vi "Map.vi"() -> ()   [LabVIEW 2010]
uses:
  Utilities/Waypoint.ctl
  Utilities/ModemTelemetryPacket.ctl
  <vilib>/Utility/sysdir.llb/System Directory Type.ctl
  <vilib>/Utility/config.llb/Write Key (String).vi
  <vilib>/Utility/config.llb/Read Key (String).vi
  <vilib>/Utility/config.llb/NI_LVConfig.lvlib
panel:
  in  "Map":refnum<k7>(container)
  out "HDOP":u16
  out "Sat Count":u16
  in  "Update Rate":dbl=5.0
  out "RSSI":u8(slide) scale=0.0..100.0
  out "Heading":u32(colorbox)=16448250
  out "Course":u32(colorbox)
  out "Capacity":u16
  out "Heading":i16
  out "Course":i16
  out "Speed":u8
  out "Altitude":dbl format="%#.1f"
  out "Longitude":dbl
  out "Latitude":dbl
  out "Battery":dbl(slide) scale=9.0..12.0 scale format="%.1f"
  out "Current":u8
  out "Voltage":dbl
  out "Compass":cluster{dbl, dbl}(knob)={0.0, 51.49737856172287} scale=0.0..360.0
  in  "Slider":bool
  out "VehiclePositionState":bool
  in  "VehicleUpdate":bool
  in  "Center":bool
  in  "Recall":bool
  in  "Load":bool
  in  "Save":bool
  in  "NoFly":bool
  in  "Home":bool
  in  "Waypoint List":T1[](array[typedef]) {"EW" items=["E", "W"]; "LonS" format="%#.1f"; "NS" items=["N", "S"]; "LatS" format="%#.1f"}
  in  "ManualAdd":bool
  in  "Up":bool
  in  "Down":bool
  in  "Delete":bool
  in  "Clear":bool
  in  "Upload":bool
  # "Lattitude"
  # "Longitude"
  # "Altitude"
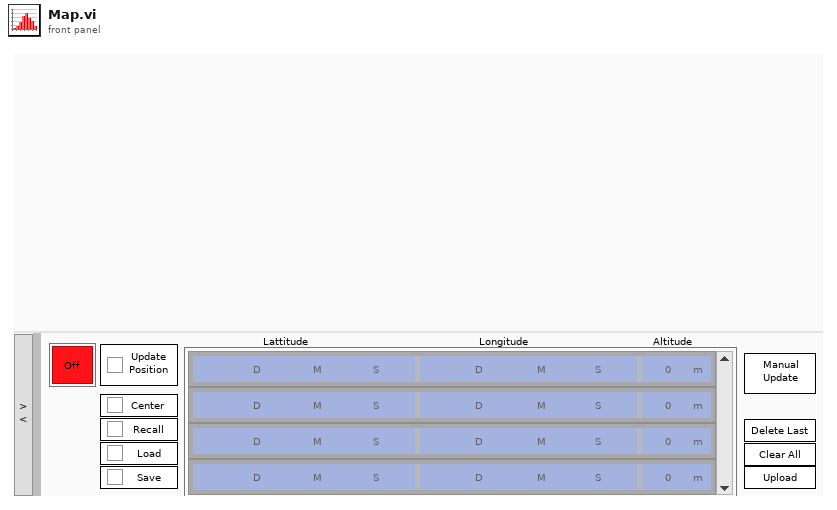
[diagram p1: front panel]
types:
  T1 = typedef "Waypoint.ctl" = cluster{"LatD":dbl, "LatM":dbl, "LatS":dbl, "LonD":dbl, "LonM":dbl, "LonS":dbl, "Alt":dbl, "NS":u16, "EW":u16}
  T2 = cluster{"Error":errorcluster, "GUIQueue":refnum<queue>, "IniData":string[][], "Map":refnum<k7>, "CookiePath":path, "Waypoints":T1[], "LastAlt":dbl, "LastType":u16, "Data":i32[][], "TlmType":string, "Compare":i32[], "Null":T1[], "MaxWaypoints":i32, "InvalidAngle":i32, "InvalidAltitude":i32, "Previous":string, "Retry":i32, "ModemQueue":refnum<queue>, "Internet":bool}
  T3 = typedef "LVRectTypeDef.ctl" = cluster{"left":i16, "top":i16, "right":i16, "bottom":i16}
  T4 = enum32{"invalid app kind", "Development System", "Run Time System", "Student Edition", "Embedded LabVIEW", "Evaluation", "Custom"}
  T5 = typedef "System Directory Type.ctl" = i32
  T6 = typedef "NI_LVConfig.lvlib/Config Data RefNum.ctl" = refnum<k1>
  T7 = enum8{"Enabled", "Disabled", "Disabled and Grayed Out"}
  T8 = typedef "ModemTelemetryPacket.ctl" = cluster{"id":u16, "latitude":i32, "longitude":i32, "altitude":i16, "course":i16, "heading":i16, "speed":u8, "voltage":u8, "current":u8, "capacity":u16, "reserved":u16, "ecc":u8[], "RSSI":u8}
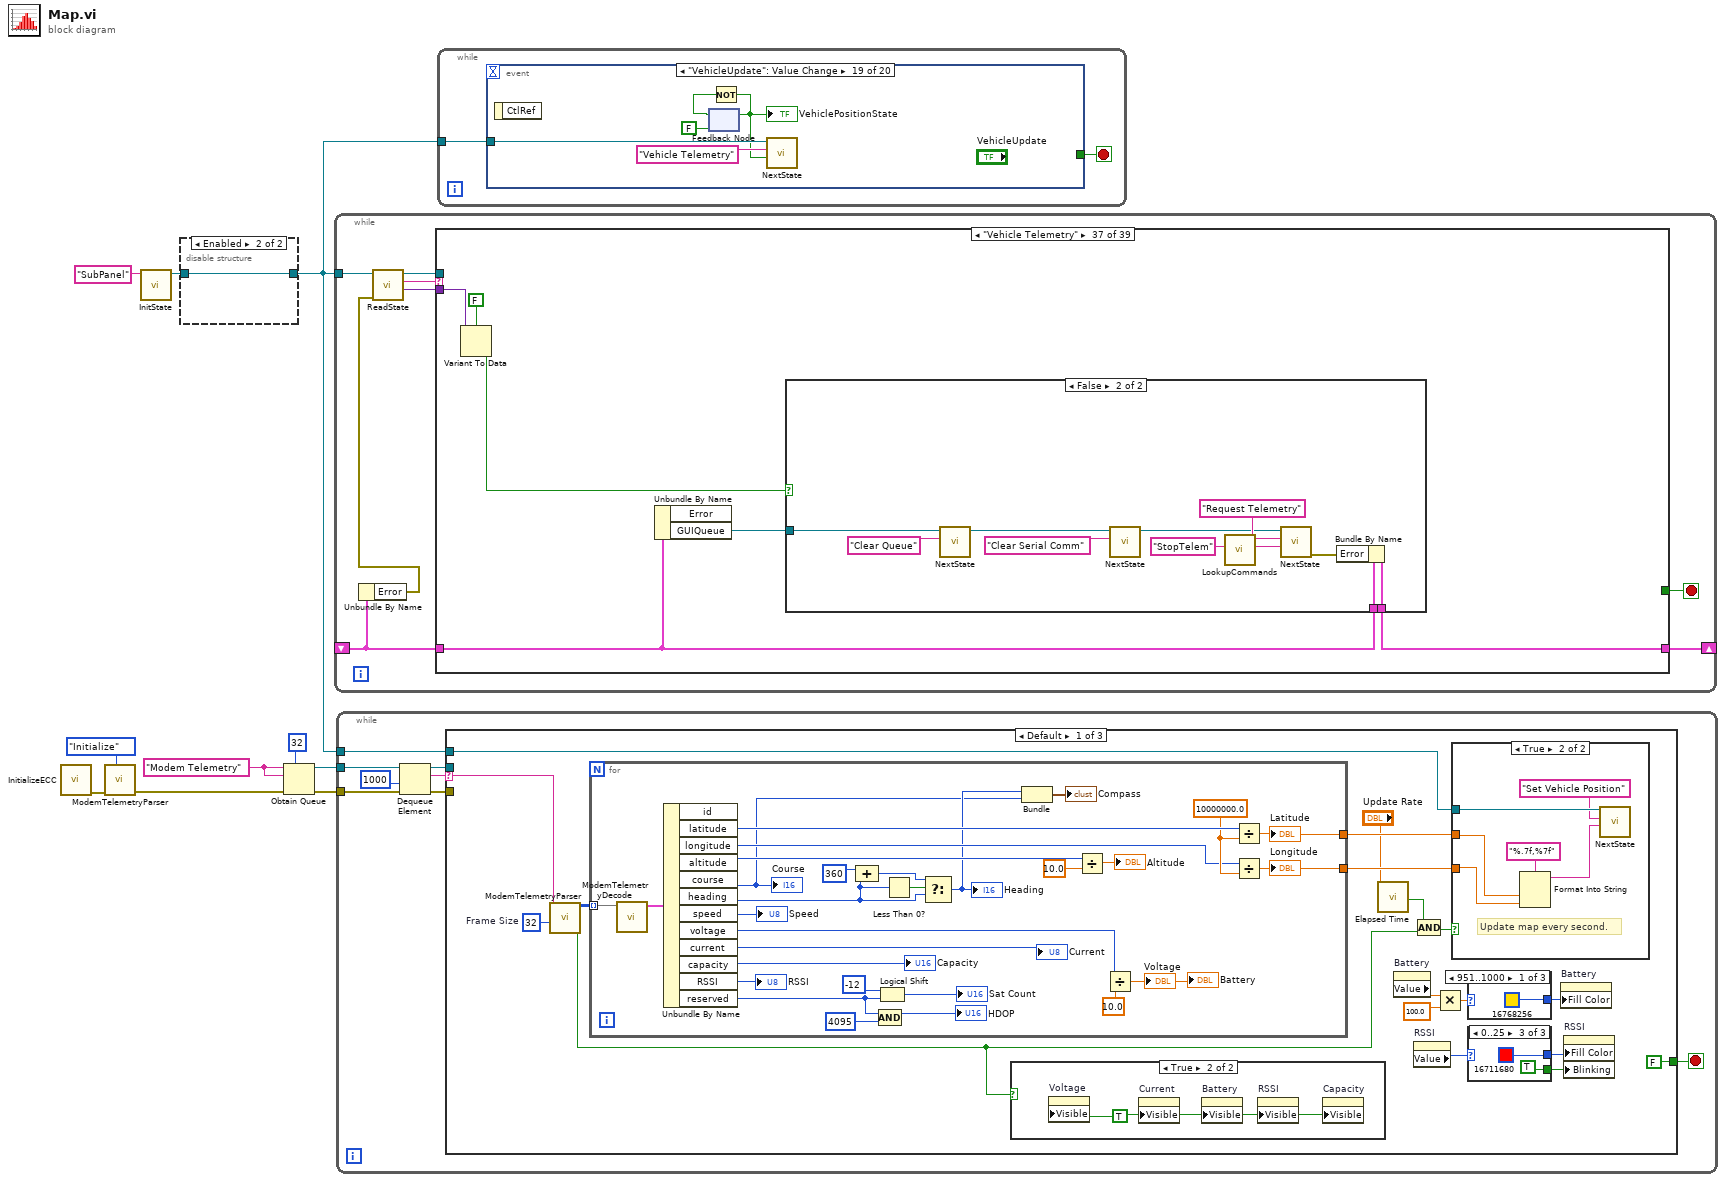
[diagram p0: block diagram]
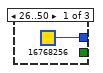
[diagram p3: hidden frame]
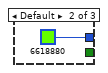
[diagram p4: hidden frame]
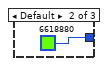
[diagram p5: hidden frame]
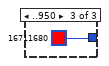
[diagram p6: hidden frame]
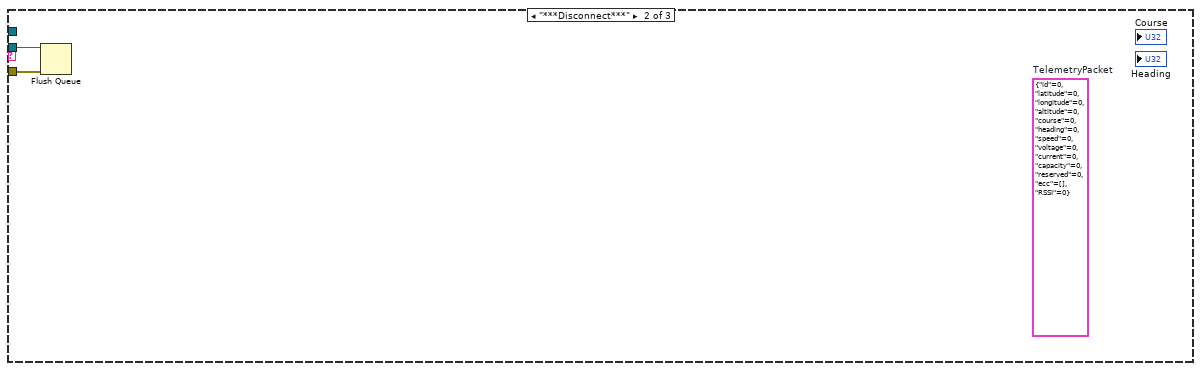
[diagram p8: hidden frame]
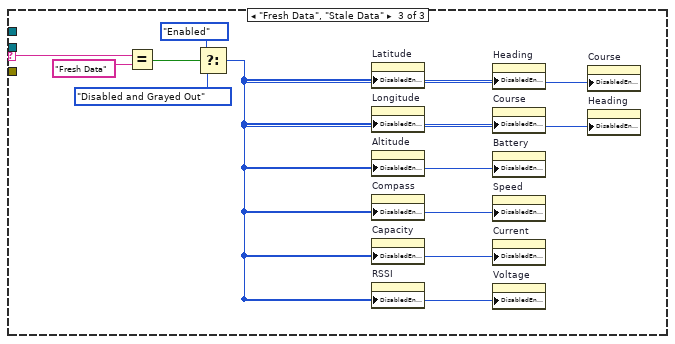
[diagram p9: hidden frame]
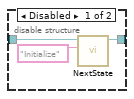
[diagram p10: hidden frame]
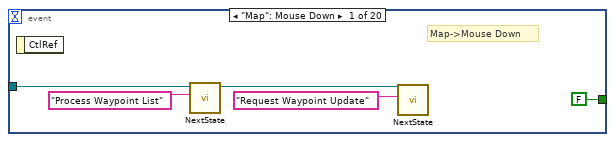
[diagram p11: hidden frame]
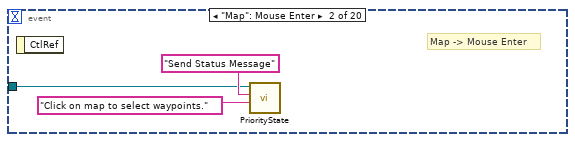
[diagram p12: hidden frame]
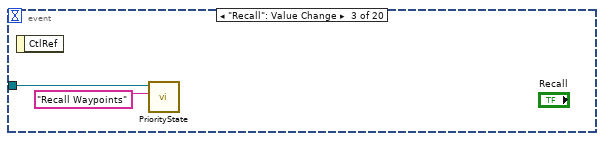
[diagram p13: hidden frame]
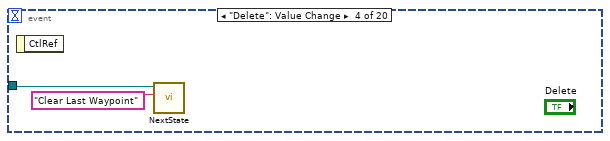
[diagram p14: hidden frame]
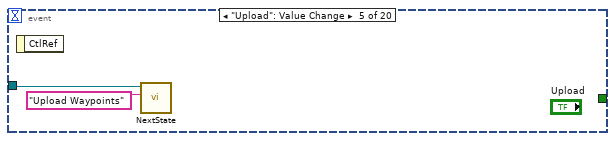
[diagram p15: hidden frame]
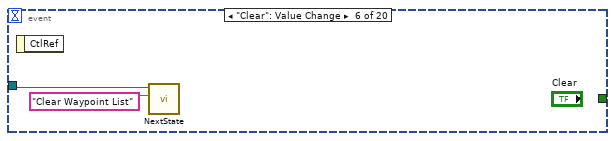
[diagram p16: hidden frame]
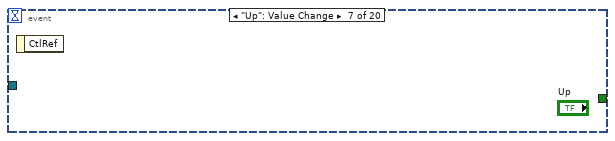
[diagram p17: hidden frame]
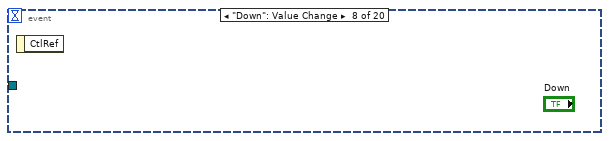
[diagram p18: hidden frame]
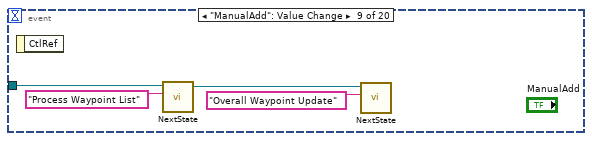
[diagram p19: hidden frame]
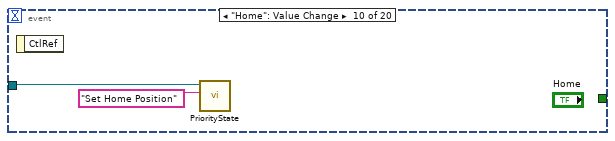
[diagram p20: hidden frame]
diagram:
  w6 = "Modem Telemetry" ("name (unnamed)")
  n1 = call "InitializeECC.vi"() -> ("Error Out"=w5:errorcluster)  [unwired: 11 in]
  n2 = call "ModemTelemetryParser.vi"("Operation"=enum16{"Parse", "Initialize"}."Initialize", "Error In"=w5) -> ("Error Out"=w4:errorcluster)  [unwired: 7 in, 2 out]
  n3 = call "InitState.vi"("Name"="SubPanel" ("name (unnamed)")) -> ("Queue Out"=w9:refnum<queue>)  [unwired: 8 in, 1 out]
  n4 = disable-structure shown="Enabled" {
    disable-tunnel: w9 -> [w13 w14]
    disable-tunnel: [w12 w14] -> w8
    frame Disabled {
      n5 = call "NextState.vi"("State"="Initialize", "Queue In"=w13) -> ("Queue Out"=w12:refnum<queue>)  [unwired: 8 in, 1 out]
    }
    frame Enabled {
    }
  }
  n6 = Obtain Queue(max queue size (-1, unlimited)=32, name (unnamed)=w6, element data type=w6, error in (no error)=w4) -> (queue out=w2:refnum<queue>, error out=w1:errorcluster)  [unwired: 1 in, 1 out]
  n7 = while {
    tunnel: w8 -> [w18]
    shift-right: [w22] -> _
    shift-left: _ -> [w21]
    stop <- w20 stop-if-true
    n8 = Unbundle By Name(w21) -> ("Error"=w19:errorcluster)
    n9 = call "ReadState.vi"("Error In"=w19, "Queue In"=w18) -> ("Data"=w15:variant, "State"=w17:string, "Queue Out"=w16:refnum<queue>)  [unwired: 6 in, 1 out]
    n10 = case shown="\"Vehicle Telemetry\"" w17 {
      tunnel: [w23 w25 w47 w55 w61 w69 w74 w98 w115 w118 w127 w128 w132 w148 w185 w200 w206 w211 w217 w227 w245 w289 w319 w334 w385 w391 w409 w421 w489 w505 w562 w572 w585 w587 w639 w721 w726 w756 w790] -> w22
      tunnel: w21 -> [w23 w25 _ w55 w62 w69 w74 w98 w115 w118 w127 w128 w132 w149 w173 w200 w206 w212 w217 w225 w245 w288 w319 w335 w385 w392 w410 w422 w489 w506 w563 w572 w585 w588 w638 w721 w727 w756 w790]
      tunnel: [_ TRUE _ _ _ _ _ _ _ _ TRUE _ _ _ _ _ _ _ _ _ _ _ _ _ _ _ _ _ _ _ _ _ _ _ _ _ _ _ _] -> w20
      tunnel: w16 -> [_ _ w42 _ _ _ _ _ _ _ _ _ w133 w156 w177 w201 _ w210 _ w223 w246 _ w321 _ w386 w394 _ w420 _ w509 _ _ _ _ w636 _ _ w753 _]
      tunnel: w15 -> [_ _ w44 w58 _ w68 _ _ _ _ _ _ _ _ _ _ _ w215 _ _ _ _ _ _ _ _ _ _ _ _ _ _ _ _ _ _ w724 _ w785]
      selector: w17 -> [_ w26 _ w57 _ _ _ _ _ _ _ _ _ _ _ _ _ _ _ _ _ _ _ _ _ _ w407 _ _ _ _ _ _ _ _ _ _ _ w786]
      frame "--- System ---" {
      }
      frame Default {
        n11 = Format Into String(format string="Invalid state:\n%s", w26) -> (resulting string=w27:string)  [unwired: 2 in, 1 out]
        n12 = One Button Dialog(message=w27) -> ()  [unwired: 1 in, 1 out]
      }
      frame "Initialize" {
        w40 = T1[] []  # Waypoints
        w37 = T2 {"Error"={"status"=FALSE, "code"=0, "source"=""}, "GUIQueue"=refnum, "IniData"=[], "Map"=refnum, "CookiePath"=path "", "Waypoints"=[], "LastAlt"=5.0, "LastType"=0, "Data"=[], "TlmType"="", "Compare"=[], "Null"=[], "MaxWaypoints"=16, "InvalidAngle"=2147483647, "InvalidAltitude"=999999999, "Previous"="", "Retry"=3, "ModemQueue"=refnum, "Internet"=FALSE}
        n13 = Variant To Data(Variant=w44, type=string[][] [] ("subarray")) -> (data=w29:string[][])  [unwired: 1 in, 1 out]
        n14 = Build Array(0) -> (w39:i32[])
        n15 = property on="Waypoint List" class="Arr (strict)"("Index Values"=w39) -> ()  [unwired: 2 in, 2 out]
        n16 = Unbundle By Name(w37) -> ("InvalidAngle"=w33:i32, "InvalidAltitude"=w32:i32, "MaxWaypoints"=w36:i32)
        n17 = call "NextStates.vi"("States"=string[] ["Read Initialization"], "Queue In"=w42) -> ()  [unwired: 8 in, 2 out]
        n18 = Bundle By Name(cluster=T1 {"LatD"=2147483647.0, "LatM"=2147483647.0, "LatS"=2147483647.0, "LonD"=2147483647.0, "LonM"=2147483647.0, "LonS"=2147483647.0, "Alt"=999999999.0, "NS"=0, "EW"=0} ("Waypoint"), "LatD"=w33, "LatM"=w33, "LatS"=w33, "LonD"=w33, "LonM"=w33, "LonS"=w33, "Alt"=w32) -> (w31:T1)
        n19 = Initialize Array(w31, w36) -> (w35:T1[])
        n20 = property class="App"() -> ("OS.Version"=w43:string)  [unwired: 2 in, 2 out]
        n21 = case shown="\"5.1\"" w43 {
          tunnel: [_ w49 w52] -> w30
          frame Default {
          }
          frame "5.1" {
            n22 = Temporary Directory() -> (w51:path)
            n23 = Build Path(base path=w51, name or relative path="..\\..\\..\\Cookies") -> (appended path=w49:path)
          }
          frame "6.1" {
            n24 = Temporary Directory() -> (w53:path)
            n25 = Build Path(base path=w53, name or relative path="..\\..\\Roaming\\Microsoft\\Windows\\Cookies") -> (appended path=w52:path)
          }
        }
        n26 = call "InitState.vi"("Name"="GUI") -> ("Queue Out"=w45:refnum<queue>)  [unwired: 8 in, 1 out]
        n27 = Bundle By Name(cluster=w37, "CookiePath"=w30, "GUIQueue"=w45, "IniData"=w29, "Null"=w35) -> (w47:T2)
        n28 = local write "Waypoint List"(w40) -> ()
      }
      frame "Send Status Message" {
        n29 = Unbundle By Name(w55) -> ("GUIQueue"=w59:refnum<queue>)
        n30 = Variant To Data(Variant=w58, type=w57) -> (data=w56:string)  [unwired: 1 in, 1 out]
        n31 = call "NextState.vi"("Data"=w56, "State"="Status", "Queue In"=w59) -> ()  [unwired: 7 in, 2 out]
      }
      frame "Error" {
        n32 = Unbundle By Name(w62) -> ("Error"=w65:errorcluster)
        n33 = call "ErrorDialog.vi"("error in"=w65) -> ("error out"=w64:errorcluster)  [unwired: 10 in]
        n34 = call <vilib>:"Clear Errors.vi"("error in (no error)"=w64) -> ("error out"=w63:errorcluster)  [unwired: 6 in]
        n35 = Bundle By Name(cluster=w62, "Error"=w63) -> (w61:T2)
      }
      frame "Delay" {
        n36 = Variant To Data(Variant=w68, type=0) -> (data=w66:i32)  [unwired: 1 in, 1 out]
        n37 = Wait (ms)(milliseconds to wait=w66) -> ()  [unwired: 1 out]
      }
      frame "Center Map" {
        n38 = Unbundle By Name(w74) -> ("Map"=w75:refnum<k7>, "Waypoints"=w72:T1[])
        n39 = Index Array(array=w72) -> (element=w73:T1)  [unwired: 1 in]
        n40 = Array Size(array=w72) -> (size(s)=w71:i32)
        n41 = Equal To 0?(x=w71) -> (x = 0?=w70:bool)
        n42 = case shown="False" w70 {
          tunnel: w75 -> [w96 _]
          tunnel: w73 -> [w79 _]
          frame False {
            n43 = Unbundle By Name(w79) -> ("NS"=w93:u16, "LatD"=w91:dbl, "LatM"=w88:dbl, "LatS"=w87:dbl, "EW"=w84:u16, "LonD"=w82:dbl, "LonM"=w81:dbl, "LonS"=w80:dbl)
            n44 = Greater Than 0?(x=w84) -> (x > 0?=w86:bool)
            n45 = Greater Than 0?(x=w93) -> (x > 0?=w92:bool)
            n46 = Negate(x=w91) -> (-x=w90:dbl)
            n47 = Negate(x=w82) -> (-x=w83:dbl)
            n48 = Select(t=w90, s=w92, f=w91) -> (s? t:f=w89:dbl)
            n49 = Select(t=w83, s=w86, f=w82) -> (s? t:f=w85:dbl)
            n50 = call "ConvertDMS2DD.vi"("Seconds"=w87, "Minutes"=w88, "Degrees"=w89) -> ("Degree Decimal"=w78:dbl)  [unwired: 7 in, 1 out]
            n51 = call "ConvertDMS2DD.vi"("Seconds"=w80, "Minutes"=w81, "Degrees"=w85) -> ("Degree Decimal"=w77:dbl)  [unwired: 7 in, 1 out]
            n52 = Format Into String(format string="javascript:centerMap(%f,%f,%d);" ("URL"), w78, w77, 17) -> (resulting string=w94:string)  [unwired: 2 in, 1 out]
            n53 = call "WaitForBrowser.vi"("BrowserCommand"=w94, "BrowserRef"=w96) -> ()  [unwired: 8 in, 2 out]
          }
          frame True {
            n54 = One Button Dialog(message="No waypoints found!  Please try loading waypoints to the AeroQuad first.") -> ()  [unwired: 1 in, 1 out]
          }
        }
      }
      frame "Move Slider" {
        n55 = property class="VI"() -> ("Front Panel.PanelBounds"=w113:T3)  [unwired: 2 in, 2 out]
        n56 = Unbundle By Name(w113) -> ("right"=w111:i16, "left"=w112:i16)
        n57 = Subtract(x=w111, y=w112) -> (x-y=w108:i16)
        n58 = property on="Splitter 5" class="Splitter"() -> ("Width"=w105:u32)  [unwired: 2 in, 2 out]
        n59 = property on="Splitter 5" class="Splitter"() -> ("Position"=w109:i32)  [unwired: 2 in, 2 out]
        n60 = property on="Slider" class="Bool"() -> ("Width"=w101:u32)  [unwired: 2 in, 2 out]
        n61 = To Unsigned Long Integer(number=w108) -> (unsigned 32bit integer=w104:u32)
        n62 = Increment(x=w105) -> (x+1=w103:u32)
        n63 = Divide(x=w108, y=2.0) -> (x/y=w106:dbl)
        n64 = Increment(x=w101) -> (x+1=w100:u32)
        n65 = Greater Or Equal?(x=w109, y=w106) -> (x >= y?=w107:bool)
        n66 = Subtract(x=w104, y=w103) -> (x-y=w102:u32)
        n67 = Select(t=w100, s=w107, f=w102) -> (s? t:f=w99:u32)
        n68 = property on="Splitter 5" class="Splitter"("Position"=w99) -> ()  [unwired: 2 in, 2 out]
      }
      frame "Move Slider Waypoint" {
        n69 = property on="Slider" class="Bool"() -> ("Width"=w116:u32)  [unwired: 2 in, 2 out]
        n70 = Increment(x=w116) -> (x+1=w114:u32)
        n71 = property on="Splitter 5" class="Splitter"("Position"=w114) -> ()  [unwired: 2 in, 2 out]
      }
      frame "Move Slider Modem" {
        n72 = property class="VI"() -> ("Front Panel.PanelBounds"=w125:T3)  [unwired: 2 in, 2 out]
        n73 = Unbundle By Name(w125) -> ("right"=w123:i16, "left"=w124:i16)
        n74 = Subtract(x=w123, y=w124) -> (x-y=w122:i16)
        n75 = property on="Splitter 5" class="Splitter"() -> ("Width"=w121:u32)  [unwired: 2 in, 2 out]
        n76 = To Unsigned Long Integer(number=w122) -> (unsigned 32bit integer=w120:u32)
        n77 = Increment(x=w121) -> (x+1=w119:u32)
        n78 = Subtract(x=w120, y=w119) -> (x-y=w117:u32)
        n79 = property on="Splitter 5" class="Splitter"("Position"=w117) -> ()  [unwired: 2 in, 2 out]
      }
      frame "Shutdown" {
      }
      frame "--- Setup ---" {
      }
      frame "Read Initialization" {
        w131 = string[] ["WaypointList", "WaypointVerify", "WriteEEPROM", "Telemetry", "StopTelem"]
        n80 = Unbundle By Name(w132) -> ("IniData"=w138:string[][], "GUIQueue"=w137:refnum<queue>)
        n81 = call "NextState.vi"("State"="Check Internet", "Queue In"=w133) -> ()  [unwired: 8 in, 2 out]
        n82 = call "NextState.vi"("Data"="Click on map to select waypoints." ("State"), "State"="Status", "Queue In"=w137) -> ()  [unwired: 7 in, 2 out]
        n83 = Index Array(array=w138, index (col)=0 ("index (row)")) -> (element=w140:string[])  [unwired: 1 in]
        n84 = for {
          tunnel: w140 -> [w146]
          tunnel: w131 -> [w142] mode=indexing
          tunnel: w138 -> [w145]
          tunnel: [w141] -> w130 mode=indexing
          n85 = Search 1D Array(1D array=w146, element=w142) -> (index of element=w143:i32)  [unwired: 1 in]
          n86 = Index Array(array=w145, index (row)=w143, index (col)=1 ("disabled index (col)")) -> (element=w141:string)
        }
        n87 = call "LookupCommands.vi"("CommandValues"=w130, "CommandNames"=w131, "Mode"=enum16{"Read", "Initialize"}."Initialize") -> ()  [unwired: 8 in, 1 out]
      }
      frame "Check Internet" {
        w155 = "74.125.127.95"  # maps.googleapis.com
        n88 = TCP Open Connection(address=w155, remote port or service name=u16 80, timeout ms (60000)=3000) -> (connection ID=w151:refnum<k5>, error out=w152:errorcluster)  [unwired: 2 in]
        n89 = TCP Close Connection(connection ID=w151, error in (no error)=w152) -> (error out=w150:errorcluster)  [unwired: 1 in, 1 out]
        n90 = case shown="No Error" w150 {
          tunnel: w156 -> [w161 w166]
          tunnel: [TRUE ("T button?") w163] -> w147
          frame No Error {
            n91 = call "NextState.vi"("Data"="Searching for stored waypoints..." ("State"), "State"="Send Status Message", "Queue In"=w161) -> ("Queue Out"=w160:refnum<queue>)  [unwired: 7 in, 1 out]
            n92 = call "NextState.vi"("State"="Load Map", "Queue In"=w160) -> ()  [unwired: 8 in, 2 out]
          }
          frame Error {
            n93 = Two Button Dialog(message="This feature requires a network connection.", 1:"Continue" ("T button name (\"OK\")"), 2:"Retry" ("T button name (\"OK\")")) -> (T button?=w163:bool)
            n94 = case shown="True" w163 {
              tunnel: w166 -> [_ w170]
              tunnel: "Check Internet" -> [_ w169]
              frame False {
              }
              frame True {
                n95 = call "NextState.vi"("State"=w169, "Queue In"=w170) -> ()  [unwired: 8 in, 2 out]
              }
            }
          }
        }
        n96 = Bundle By Name(cluster=w149, "Internet"=w147) -> (w148:T2)
      }
      frame "Load Map" {
        (unwired) "Ask User To Recall Waypoints" ("State")
        n97 = call "NextState.vi"("State"="Recall Waypoints", "Queue In"=w177) -> ()  [unwired: 8 in, 2 out]
        n98 = property class="App"() -> ("App.Kind"=w184:T4)  [unwired: 2 in, 2 out]
        n99 = property class="App"() -> ("OS.Name"=w182:string)  [unwired: 2 in, 2 out]
        n100 = call <userlib>:"Current VIs Parent Directory__ogtk.vi"() -> ("Parent Directory (+ Relative)"=w183:path)  [unwired: 5 in]
        n101 = case shown="\"Run Time System\", Default" w184 {
          tunnel: [w190 w198] -> w180
          tunnel: w183 -> [w193 w198]
          tunnel: w182 -> [w191 _]
          frame "Run Time System", Default {
            n102 = case shown="\"Mac OS\"" w191 {
              tunnel: [w195 w197] -> w194
              tunnel: w193 -> [w195 w196]
              frame Default {
              }
              frame "Mac OS" {
                n103 = Strip Path(path=w196) -> (stripped path=w197:path)  [unwired: 1 out]
              }
            }
            n104 = Build Path(base path=w194, name or relative path=path "Support") -> (appended path=w190:path)
          }
          frame "Development System" {
          }
        }
        n105 = Unbundle By Name(w173) -> ("Internet"=w172:bool)
        n106 = Build Path(base path=w180, name or relative path="AeroQuad.cfg") -> (appended path=w181:path)
        n107 = Path To String(path=w181) -> (string=w179:string)
        n108 = call "WaitForBrowser.vi"("Connection"=w172, "BrowserCommand"=w179, "BrowserRef"="Map") -> ("BrowserRefOut"=w175:refnum<k7>)  [unwired: 7 in, 1 out]
        n109 = disable-structure shown="Disabled" {
          disable-tunnel: w175 -> [w188 w189]
          disable-tunnel: [w187 w189] -> w174
          frame Disabled {
            n110 = call "WaitForBrowser.vi"("BrowserCommand"="javascript:showVehicle(true);", "BrowserRef"=w188) -> ("BrowserRefOut"=w187:refnum<k7>)  [unwired: 8 in, 1 out]
          }
          frame Enabled {
          }
        }
        n111 = Bundle By Name(cluster=w173, "Map"=w174) -> (w185:T2)
      }
      frame "Ask User To Recall Waypoints" {
        n112 = Two Button Dialog(message="Would you like to recall waypoints stored in the AeroQuad?\n\nYou must be connected to the AeroQuad to complete this operation.  Waypoints can be recalled at any time by selecting the \"Recall\" button. ") -> (T button?=w202:bool)  [unwired: 2 in]
        n113 = case shown="True" w202 {
          tunnel: w201 -> [_ w204]
          frame False {
          }
          frame True {
            n114 = call "NextState.vi"("State"="Recall Waypoints", "Queue In"=w204) -> ()  [unwired: 8 in, 2 out]
          }
        }
      }
      frame "Set Home Position" {
        n115 = Unbundle By Name(w206) -> ("Map"=w205:refnum<k7>)
        n116 = flat-sequence {
          tunnel: w205 -> [w207]
          frame #0 {
            n117 = invoke class="IWebBrowser2" method="Navigate"(reference=w207, "URL"="javascript:clearMap();") -> ()  [unwired: 6 in, 8 out]
            n118 = One Button Dialog(message="Click on your desired default start position.") -> ()  [unwired: 1 in, 1 out]
          }
          frame #1 {
            # "Retrieve Waypoint"
          }
          frame #2 {
            # "Store to Disk"
          }
          frame #3 {
            # "Center Map"
          }
        }
      }
      frame "Update" {
        # "When initializing for the type of\ncalibration / telemetry, populate\nTlmType with the state where\nthis data will be processed as\nreceived from main Configurator."
        n119 = Variant To Data(Variant=w215, type=i32[][] []) -> (data=w213:i32[][])  [unwired: 1 in, 1 out]
        n120 = Bundle By Name(cluster=w212, "Data"=w213) -> (w211:T2)
        n121 = Unbundle By Name(w211) -> ("TlmType"=w214:string)
        n122 = call "NextState.vi"("State"=w214, "Queue In"=w210) -> ()  [unwired: 8 in, 2 out]
      }
      frame "--- Configure Waypoints ---" {
      }
      frame "Process Waypoint List" {
        n123 = Unbundle By Name(w225) -> ("MaxWaypoints"=w221:i32)
        n124 = Array Size(array="Waypoint List") -> (size(s)=w224:i32)
        n125 = Greater Or Equal?(x=w224, y=w221) -> (x >= y?=w222:bool)
        n126 = Decrement(x=w224) -> (x-1=w218:i32)
        n127 = Index Array(array="Waypoint List", index=w218) -> (element=w219:T1)
        n128 = Unbundle By Name(w219) -> ("Alt"=w220:dbl)
        n129 = case shown="..-1" w218 {
          tunnel: w220 -> [_ w235]
          tunnel: w225 -> [w230 w234]
          tunnel: "Waypoint List" -> [w228 w233]
          tunnel: [w229 w232] -> w227
          frame ..-1 {
            w231 = u16 0  # Future Use
            n130 = Bundle By Name(cluster=w230, "Waypoints"=w228, "LastType"=w231) -> (w229:T2)
          }
          frame Default {
            w236 = u16 0  # Future Use
            n131 = Bundle By Name(cluster=w234, "Waypoints"=w233, "LastType"=w236, "LastAlt"=w235) -> (w232:T2)
          }
        }
        n132 = case shown="False" w222 {
          tunnel: w223 -> [_ w238]
          tunnel: w221 -> [_ w237]
          frame False {
          }
          frame True {
            n133 = Format Into String(format string="Maximum number of %d waypoints has been reached! ", w237) -> (resulting string=w242:string)  [unwired: 2 in, 1 out]
            n134 = call "NextState.vi"("Data"=w242, "State"="Send Status Message" ("format string"), "Queue In"=w238) -> ("Queue Out"=w243:refnum<queue>)  [unwired: 7 in, 1 out]
            n135 = call "NextState.vi"("State"="Clear Last Waypoint", "Queue In"=w243) -> ()  [unwired: 8 in, 2 out]
          }
        }
      }
      frame "Manual Waypoint Update" {
        n136 = local read "Waypoint List"() -> (w249:T1[])
        n137 = Unbundle By Name(w245) -> ("Waypoints"=w248:T1[], "Internet"=w244:bool)
        n138 = Equal?(x=w249, y=w248) -> (x = y?=w247:bool)
        n139 = case shown="False" w247 {
          tunnel: w245 -> [w277 _]
          tunnel: w249 -> [w276 _]
          tunnel: w246 -> [w275 _]
          tunnel: w244 -> [w250 _]
          frame False {
            # "Add last waypoint in the list"
            n140 = Array Size(array=w276) -> (size(s)=w273:i32)
            n141 = Decrement(x=w273) -> (x-1=w278:i32)
            n142 = Index Array(array=w276, index=w278) -> (element=w251:T1)
            n143 = Unbundle By Name(w251) -> ("NS"=w272:u16, "LatD"=w270:dbl, "LatM"=w267:dbl, "LatS"=w266:dbl, "EW"=w263:u16, "LonD"=w261:dbl, "LonM"=w260:dbl, "LonS"=w259:dbl)
            n144 = call "PriorityState.vi"("State"="Request Waypoint Update", "Queue In"=w275) -> ()  [unwired: 8 in, 2 out]
            n145 = Greater Than 0?(x=w263) -> (x > 0?=w265:bool)
            n146 = Greater Than 0?(x=w272) -> (x > 0?=w271:bool)
            n147 = Negate(x=w270) -> (-x=w269:dbl)
            n148 = Negate(x=w261) -> (-x=w262:dbl)
            n149 = Select(t=w269, s=w271, f=w270) -> (s? t:f=w268:dbl)
            n150 = Select(t=w262, s=w265, f=w261) -> (s? t:f=w264:dbl)
            n151 = call "ConvertDMS2DD.vi"("Seconds"=w266, "Minutes"=w267, "Degrees"=w268) -> ("Degree Decimal"=w257:dbl)  [unwired: 7 in, 1 out]
            n152 = call "ConvertDMS2DD.vi"("Seconds"=w259, "Minutes"=w260, "Degrees"=w264) -> ("Degree Decimal"=w256:dbl)  [unwired: 7 in, 1 out]
            n153 = Number To Fractional String(number=w257) -> (F-format string=w254:string)  [unwired: 3 in]
            n154 = Number To Fractional String(number=w256) -> (F-format string=w253:string)  [unwired: 3 in]
            n155 = Concatenate Strings(w254, "," ("string"), w253) -> (w255:string)
            n156 = Format Into String(format string="javascript:setManualWaypoint(%s);" ("URL"), w255) -> (resulting string=w279:string)  [unwired: 2 in, 1 out]
            n157 = Unbundle By Name(w277) -> ("Map"=w280:refnum<k7>)
            n158 = call "WaitForBrowser.vi"("Connection"=w250, "BrowserCommand"=w279, "BrowserRef"=w280) -> ()  [unwired: 7 in, 2 out]
          }
          frame True {
          }
        }
      }
      frame "Overall Waypoint Update" {
        # "add all waypoints in list to map"
        # "Update complete waypoint list."
        n159 = Unbundle By Name(w288) -> ("Waypoints"=w287:T1[], "Map"=w285:refnum<k7>, "Internet"=w281:bool)
        n160 = call "WaitForBrowser.vi"("Connection"=w281, "BrowserCommand"="javascript:clearMap();" ("URL"), "BrowserRef"=w285) -> ("Error Out"=w283:errorcluster, "BrowserRefOut"=w286:refnum<k7>)  [unwired: 7 in]
        n161 = for {
          tunnel: w287 -> [w295] mode=indexing
          shift-right: [w292] -> w282
          shift-left: w283 -> [w291]
          tunnel: w286 -> [w293]
          tunnel: w281 -> [w290]
          n162 = Unbundle By Name(w295) -> ("NS"=w316:u16, "LatD"=w314:dbl, "LatM"=w311:dbl, "LatS"=w310:dbl, "EW"=w307:u16, "LonD"=w305:dbl, "LonM"=w304:dbl, "LonS"=w303:dbl)
          n163 = Greater Than 0?(x=w307) -> (x > 0?=w309:bool)
          n164 = Greater Than 0?(x=w316) -> (x > 0?=w315:bool)
          n165 = Negate(x=w314) -> (-x=w313:dbl)
          n166 = Negate(x=w305) -> (-x=w306:dbl)
          n167 = Select(t=w313, s=w315, f=w314) -> (s? t:f=w312:dbl)
          n168 = Select(t=w306, s=w309, f=w305) -> (s? t:f=w308:dbl)
          n169 = call "ConvertDMS2DD.vi"("Seconds"=w310, "Minutes"=w311, "Degrees"=w312) -> ("Degree Decimal"=w301:dbl)  [unwired: 7 in, 1 out]
          n170 = call "ConvertDMS2DD.vi"("Seconds"=w303, "Minutes"=w304, "Degrees"=w308) -> ("Degree Decimal"=w300:dbl)  [unwired: 7 in, 1 out]
          n171 = Number To Fractional String(number=w301) -> (F-format string=w298:string)  [unwired: 3 in]
          n172 = Number To Fractional String(number=w300) -> (F-format string=w297:string)  [unwired: 3 in]
          n173 = Concatenate Strings(w298, "," ("string"), w297) -> (w299:string)
          n174 = Format Into String(format string="javascript:setManualWaypoint(%s);" ("URL"), w299) -> (resulting string=w294:string)  [unwired: 2 in, 1 out]
          n175 = call "WaitForBrowser.vi"("Connection"=w290, "BrowserCommand"=w294, "Error In"=w291, "BrowserRef"=w293) -> ("Error Out"=w292:errorcluster)  [unwired: 6 in, 1 out]
        }
        n176 = Bundle By Name(cluster=w288, "Waypoints"=w287, "Error"=w282) -> (w289:T2)
      }
      frame "Request Waypoint Update" {
        n177 = call "PriorityState.vi"("State"="Update Waypoint List", "Queue In"=w321) -> ()  [unwired: 8 in, 2 out]
        n178 = Unbundle By Name(w319) -> ("Map"=w323:refnum<k7>, "Internet"=w317:bool)
        n179 = call "WaitForBrowser.vi"("Connection"=w317, "BrowserCommand"="javascript:queryWaypointList();" ("URL"), "BrowserRef"=w323) -> ("Error Out"=w318:errorcluster)  [unwired: 7 in, 1 out]
        n180 = call "Time Delay"("error in (no error)"=w318) -> ()  [unwired: 10 in, 1 out]
      }
      frame "Update Waypoint List" {
        n181 = Unbundle By Name(w335) -> ("CookiePath"=w361:path)
        n182 = List Folder(path=w361) -> (path out=w360:path, filenames=w359:string[])  [unwired: 3 in, 2 out]
        n183 = for {
          tunnel: w360 -> [w383]
          tunnel: w359 -> [w382] mode=indexing
          tunnel: [w380] -> w352 mode=indexing
          tunnel: [w379] -> w356 mode=indexing
          n184 = Build Path(base path=w383, name or relative path=w382) -> (appended path=w381:path)
          n185 = File/Directory Info(path=w381) -> (path out=w379:path, last mod=w380:timestamp)  [unwired: 1 in, 5 out]
        }
        n186 = Sort 1D Array(array=w352) -> (sorted array=w355:timestamp[])
        n187 = Array Size(array=w355) -> (size(s)=w358:i32)
        n188 = Unbundle By Name(w335) -> ("Waypoints"=w326:T1[], "LastAlt"=w340:dbl, "LastType"=w341:u16)
        n189 = Decrement(x=w358) -> (x-1=w357:i32)
        n190 = Index Array(array=w355, index=w357) -> (element=w354:timestamp)
        n191 = Search 1D Array(1D array=w352, element=w354) -> (index of element=w353:i32)  [unwired: 1 in]
        n192 = Index Array(array=w356, index=w353) -> (element=w325:path)
        n193 = Array Size(array=w326) -> (size(s)=w333:i32)
        n194 = Read from Text File(file (use dialog)=w325) -> (text=w351:string)  [unwired: 3 in, 3 out]
        n195 = Match Pattern(string=w351, regular expression="{{") -> (after substring=w349:string)  [unwired: 1 in, 3 out]
        n196 = Match Pattern(string=w349, regular expression="}}") -> (before substring=w324:string)  [unwired: 1 in, 3 out]
        n197 = Search and Replace String(replace all?=TRUE ("replace all? (F)"), input string=w324, search string="(") -> (result string=w344:string)  [unwired: 5 in, 3 out]
        n198 = Spreadsheet String To Array(delimiter (Tab)=")", format string="%s", spreadsheet string=w344, array type (2D Dbl)=string[] []) -> (array=w339:string[])
        n199 = Array Size(array=w339) -> (size(s)=w337:i32)
        n200 = Decrement(x=w337) -> (x-1=w338:i32)
        n201 = for {
          N: w338 -> [_]
          tunnel: w339 -> [w372] mode=indexing
          tunnel: [w371] -> w327 mode=indexing
          tunnel: w341 -> [w368]
          tunnel: w340 -> [w363]
          tunnel: [w367] -> w329
          tunnel: w326 -> [w369]
          tunnel: w333 -> [w370]
          tunnel: [w366] -> w332
          tunnel: [w365] -> w331
          i -> [w367]
          n202 = Greater Or Equal?(x=w367, y=w370) -> (x >= y?=w364:bool)
          n203 = case shown="False" w364 {
            tunnel: w369 -> [w375 _]
            tunnel: w367 -> [w376 _]
            tunnel: [w373 w378] -> w366
            tunnel: [_ w377] -> w365
            tunnel: w363 -> [_ w378]
            tunnel: w368 -> [_ w377]
            frame False {
              n204 = Index Array(array=w375, index=w376) -> (element=w374:T1)
              n205 = Unbundle By Name(w374) -> ("Alt"=w373:dbl)
            }
            frame True {
            }
          }
          n206 = call "CreateWaypoint.vi"("Use Default?"=TRUE, "Altitude"=w366, "Coordinates"=w372, "Type"=w365) -> ("Waypoint"=w371:T1)  [unwired: 7 in]
        }
        n207 = local write "Waypoint List"(w327) -> ()
        n208 = Subtract(x=w329, y=2) -> (x-y=w330:i32)
        n209 = Build Array(w330) -> (w336:i32[])
        n210 = property on="Waypoint List" class="Arr (strict)"("Index Values"=w336) -> ()  [unwired: 2 in, 2 out]
        n211 = Bundle By Name(cluster=w335, "LastAlt"=w332, "LastType"=w331, "Waypoints"=w327) -> (w334:T2)
      }
      frame "Clear Last Waypoint" {
        n212 = call "PriorityState.vi"("State"="Request Waypoint Update", "Queue In"=w386) -> ()  [unwired: 8 in, 2 out]
        n213 = Unbundle By Name(w385) -> ("Map"=w389:refnum<k7>, "Internet"=w384:bool)
        n214 = call "WaitForBrowser.vi"("Connection"=w384, "BrowserCommand"="javascript:clearLastWaypoint();" ("URL"), "BrowserRef"=w389) -> ()  [unwired: 7 in, 2 out]
      }
      frame "Clear Waypoint List" {
        w393 = T1[] []  # Waypoints
        n215 = Unbundle By Name(w392) -> ("Map"=w397:refnum<k7>, "Internet"=w390:bool)
        n216 = call "PriorityState.vi"("State"="Request Waypoint Update", "Queue In"=w394) -> ()  [unwired: 8 in, 2 out]
        n217 = call "WaitForBrowser.vi"("Connection"=w390, "BrowserCommand"="javascript:clearMap();" ("URL"), "BrowserRef"=w397) -> ()  [unwired: 7 in, 2 out]
        n218 = local write "Waypoint List"(w393) -> ()
        n219 = Bundle By Name(cluster=w392, "Waypoints"=w393) -> (w391:T2)
      }
      frame "Recall Waypoints" {
        n220 = Unbundle By Name(w410) -> ("GUIQueue"=w404:refnum<queue>)
        n221 = call "NextState.vi"("Data"="Searching for stored waypoints on the AeroQuad." ("State"), "State"="Status", "Queue In"=w404) -> ("Queue Out"=w406:refnum<queue>)  [unwired: 7 in, 1 out]
        n222 = call "LookupCommands.vi"("CommandName"="WaypointVerify") -> ("CommandValue"=w412:string)  [unwired: 10 in]
        n223 = call "NextState.vi"("Data"=w412, "State"="Request Telemetry", "Queue In"=w406) -> ("Queue Out"=w401:refnum<queue>)  [unwired: 7 in, 1 out]
        n224 = call "NextState.vi"("Data"=500, "State"="Delay", "Queue In"=w401) -> ("Queue Out"=w400:refnum<queue>)  [unwired: 7 in, 1 out]
        n225 = call "NextState.vi"("State"="Read Integers Once", "Queue In"=w400) -> ()  [unwired: 8 in, 2 out]
        n226 = property on="Waypoint List" class="Arr (strict)"("Index Values"=u32[] [0]) -> ()  [unwired: 2 in, 2 out]
        n227 = Bundle By Name(cluster=w410, "Previous"=w407, "TlmType"="Update Recalled Waypoints") -> (w409:T2)
      }
      frame "Update Recalled Waypoints" {
        n228 = Unbundle By Name(w422) -> ("Data"=w419:i32[][], "Previous"=w416:string, "Retry"=w415:i32)
        n229 = Array Size(array=w419) -> (size(s)=w418:i32[])
        n230 = Index Array(array=w418) -> (element=w417:i32)  [unwired: 1 in]
        n231 = case shown="0" w417 {
          tunnel: w422 -> [w429 w453]
          tunnel: [w428 w452] -> w421
          tunnel: w420 -> [w431 w437]
          tunnel: w419 -> [_ w440]
          tunnel: w416 -> [w430 _]
          tunnel: w415 -> [w425 _]
          frame 0 {
            n232 = Greater Or Equal?(x=w425, y=3) -> (x >= y?=w426:bool)
            n233 = Increment(x=w425) -> (x+1=w424:i32)
            n234 = case shown="True" w426 {
              tunnel: w431 -> [w434 _]
              tunnel: w430 -> [w433 _]
              tunnel: w424 -> [w432 _]
              tunnel: [w432 _] -> w423
              frame False {
                n235 = call "NextState.vi"("State"=w433, "Queue In"=w434) -> ()  [unwired: 8 in, 2 out]
              }
              frame True {
                n236 = One Button Dialog(message="Unable to recall waypoints.\nPlease try again.") -> ()  [unwired: 1 in, 1 out]
              }
            }
            n237 = Bundle By Name(cluster=w429, "Retry"=w423) -> (w428:T2)
          }
          frame Default {
            n238 = Index Array(array=w440) -> (element=w457:i32[])  [unwired: 2 in]
            n239 = Reshape Array(w457, 16 ("dimension size"), 4 ("dimension size")) -> (w446:i32[][])
            n240 = Index Array(array=w446, index (col)=1 ("disabled index (col)")) -> (element=w445:i32[])  [unwired: 1 in]
            n241 = Search 1D Array(1D array=w445, element=2147483647) -> (index of element=w443:i32)  [unwired: 1 in]
            n242 = call "NextState.vi"("State"="Overall Waypoint Update", "Queue In"=w437) -> ("Queue Out"=w436:refnum<queue>)  [unwired: 8 in, 1 out]
            n243 = for {
              N: w443 -> [_]
              tunnel: w446 -> [w487] mode=indexing
              tunnel: T1 {"LatD"=0.0, "LatM"=0.0, "LatS"=0.0, "LonD"=0.0, "LonM"=0.0, "LonS"=0.0, "Alt"=0.0, "NS"=0, "EW"=0} ("Waypoint") -> [w488]
              tunnel: [w463] -> w442 mode=indexing
              w461 = FALSE ("Type")
              w464 = u16 1 items=["E", "W"] ("EW")
              w465 = u16 0 items=["E", "W"] ("EW")
              w470 = u16 1 items=["N", "S"] ("NS")
              w471 = u16 0 items=["N", "S"] ("NS")
              n244 = Index Array(array=w487, index #1=1 ("index")) -> (element #1=w486:i32, element #2=w480:i32, element #3=w478:i32)  [unwired: 2 in]
              n245 = To Double Precision Float(number=w486) -> (double precision float=w483:dbl)
              n246 = To Double Precision Float(number=w480) -> (double precision float=w482:dbl)
              n247 = To Double Precision Float(number=w478) -> (double precision float=w460:dbl)
              n248 = Divide(x=w483, y=10000000.0) -> (x/y=w484:dbl)
              n249 = Divide(x=w482, y=10000000.0) -> (x/y=w479:dbl)
              n250 = Divide(x=w460, y=100.0) -> (x/y=w459:dbl)
              n251 = call "ConvertDD2DMS.vi"("Type"=w461, "Degree Decimal"=w484) -> ("Seconds"=w475:dbl, "Minutes"=w476:dbl, "Degrees"=w477:dbl, "NE?"=w472:bool)  [unwired: 5 in, 1 out]
              n252 = call "ConvertDD2DMS.vi"("Type"=w461, "Degree Decimal"=w479) -> ("Seconds"=w473:dbl, "Minutes"=w474:dbl, "Degrees"=w468:dbl, "NE?"=w467:bool)  [unwired: 5 in, 1 out]
              n253 = Select(t=w471, s=w472, f=w470) -> (s? t:f=w469:u16)
              n254 = Select(t=w465, s=w467, f=w464) -> (s? t:f=w466:u16)
              n255 = Bundle By Name(cluster=w488, "LatD"=w477, "LatM"=w476, "LatS"=w475, "NS"=w469, "LonD"=w468, "LonM"=w474, "LonS"=w473, "EW"=w466, "Alt"=w459) -> (w463:T1)
            }
            n256 = call "NextState.vi"("State"="Center Map", "Queue In"=w436) -> ()  [unwired: 8 in, 2 out]
            n257 = Array Size(array=w442) -> (size(s)=w448:i32)
            n258 = local write "Waypoint List"(w442) -> ()
            n259 = Bundle By Name(cluster=w453, "Waypoints"=w442, "Retry"=0) -> (w452:T2)
            n260 = Subtract(x=w448, y=3) -> (x-y=w450:i32)
            n261 = Build Array(w450) -> (w451:i32[])
            n262 = property on="Waypoint List" class="Arr (strict)"("Index Values"=w451) -> ()  [unwired: 2 in, 2 out]
          }
        }
      }
      frame "--- Upload ---" {
      }
      frame "Upload Waypoints" {
        n263 = Unbundle By Name(w506) -> ("MaxWaypoints"=w501:i32, "Waypoints"=w503:T1[])
        n264 = Unbundle By Name(w506) -> ("Null"=w504:T1[], "GUIQueue"=w499:refnum<queue>)
        n265 = Replace Array Subset(array=w504, new element=w503) -> (w502:T1[])  [unwired: 1 in]
        n266 = call "NextState.vi"("State"="Verify Upload", "Queue In"=w509) -> ()  [unwired: 8 in, 2 out]
        n267 = call "NextState.vi"("Data"="Uploading waypoints, please wait..." ("State"), "State"="Status", "Queue In"=w499) -> ("Queue Out"=w500:refnum<queue>)  [unwired: 7 in, 1 out]
        n268 = call "LookupCommands.vi"("CommandName"="WaypointList") -> ("CommandValue"=w510:string)  [unwired: 10 in]
        n269 = for {
          N: w501 -> [_]
          tunnel: w502 -> [w551] mode=indexing
          tunnel: w500 -> [w549]
          tunnel: w510 -> [w545]
          shift-right: [w542] -> w507
          shift-left: i32[] [] -> [w543]
          tunnel: [w517] -> w495
          i -> [w538]
          n270 = Unbundle By Name(w551) -> ("NS"=w537:u16, "LatD"=w535:dbl, "LatM"=w532:dbl, "LatS"=w531:dbl, "EW"=w528:u16, "LonD"=w526:dbl, "LonM"=w525:dbl, "LonS"=w524:dbl, "Alt"=w515:dbl)
          n271 = Greater Than 0?(x=w528) -> (x > 0?=w530:bool)
          n272 = Greater Than 0?(x=w537) -> (x > 0?=w536:bool)
          n273 = Negate(x=w535) -> (-x=w534:dbl)
          n274 = Negate(x=w526) -> (-x=w527:dbl)
          n275 = Select(t=w534, s=w536, f=w535) -> (s? t:f=w533:dbl)
          n276 = Select(t=w527, s=w530, f=w526) -> (s? t:f=w529:dbl)
          n277 = call "ConvertDMS2DD.vi"("Seconds"=w531, "Minutes"=w532, "Degrees"=w533) -> ("Degree Decimal"=w523:dbl)  [unwired: 7 in, 1 out]
          n278 = call "ConvertDMS2DD.vi"("Seconds"=w524, "Minutes"=w525, "Degrees"=w529) -> ("Degree Decimal"=w520:dbl)  [unwired: 7 in, 1 out]
          n279 = Compound Arithmetic op=MULTIPLY(w515, 100.0 ("value")) -> (w514:dbl)
          n280 = Compound Arithmetic op=MULTIPLY(w523, 10000000.0) -> (w518:dbl)
          n281 = Compound Arithmetic op=MULTIPLY(w520, 10000000.0) -> (w519:dbl)
          n282 = To Long Integer(number=w514) -> (32bit integer=w541:i32)
          n283 = To Long Integer(number=w518) -> (32bit integer=w539:i32)
          n284 = To Long Integer(number=w519) -> (32bit integer=w540:i32)
          n285 = Format Into String(format string="%d;%d;%d;%d;", initial string=w545, w538, w539, w540, w541) -> (resulting string=w544:string)  [unwired: 1 in, 1 out]
          n286 = call "NextState.vi"("Data"=w544, "State"="Send Command", "Queue In"=w549) -> ("Queue Out"=w547:refnum<queue>)  [unwired: 7 in, 1 out]
          n287 = Build Array (concatenate)(w543, w538, w539, w540, w541) -> (w542:i32[])
          n288 = call "NextState.vi"("Data"=250, "State"="Delay", "Queue In"=w547) -> ("Queue Out"=w517:refnum<queue>)  [unwired: 7 in, 1 out]
        }
        n289 = call "LookupCommands.vi"("CommandName"="WriteEEPROM") -> ("CommandValue"=w493:string)  [unwired: 10 in]
        n290 = call "NextState.vi"("Data"=w493, "State"="Send Command", "Queue In"=w495) -> ("Queue Out"=w490:refnum<queue>)  [unwired: 7 in, 1 out]
        n291 = Bundle By Name(cluster=w506, "Compare"=w507) -> (w505:T2)
        n292 = call "NextState.vi"("Data"=1000, "State"="Delay", "Queue In"=w490) -> ()  [unwired: 7 in, 2 out]
      }
      frame "Verify Upload" {
        n293 = Unbundle By Name(w563) -> ("GUIQueue"=w557:refnum<queue>)
        n294 = call "NextState.vi"("Data"="Verifying waypoint upload..." ("State"), "State"="Status", "Queue In"=w557) -> ("Queue Out"=w556:refnum<queue>)  [unwired: 7 in, 1 out]
        n295 = call "LookupCommands.vi"("CommandName"="WaypointVerify") -> ("CommandValue"=w564:string)  [unwired: 10 in]
        n296 = call "NextState.vi"("Data"=w564, "State"="Request Telemetry", "Queue In"=w556) -> ("Queue Out"=w555:refnum<queue>)  [unwired: 7 in, 1 out]
        n297 = call "NextState.vi"("Data"=500, "State"="Delay", "Queue In"=w555) -> ("Queue Out"=w554:refnum<queue>)  [unwired: 7 in, 1 out]
        n298 = call "NextState.vi"("State"="Read Integers Once", "Queue In"=w554) -> ()  [unwired: 8 in, 2 out]
        n299 = Bundle By Name(cluster=w563, "TlmType"="Verify Waypoints") -> (w562:T2)
      }
      frame "Verify Waypoints" {
        n300 = Unbundle By Name(w572) -> ("GUIQueue"=w570:refnum<queue>, "Data"=w571:i32[][], "Compare"=w567:i32[])
        n301 = Index Array(array=w571) -> (element=w568:i32[])  [unwired: 2 in]
        n302 = Equal?(x=w568, y=w567) -> (x = y?=w569:bool)
        n303 = case shown="True" w569 {
          tunnel: w570 -> [_ w582]
          tunnel: w568 -> [w578 _]
          tunnel: w567 -> [w577 _]
          frame False {
            w575 = "," ("delimiter (Tab)")
            w576 = "%d" ("format string")
            n304 = Array To Spreadsheet String(delimiter (Tab)=w575, array=w578, 3:w576) -> (spreadsheet string=w574:string)
            n305 = Array To Spreadsheet String(delimiter (Tab)=w575, array=w577, 3:w576) -> (spreadsheet string=w573:string)
            n306 = Format Into String(format string="Error in verifying waypoint upload!\n\nRetrieved waypoints:\n%s\nExpected waypoints:\n%s\n\nPlease retry waypoint upload.  If after retrying the upload, you still experience errors, please disconnect the AeroQuad and retry again as the messages maybe out of sync.", w574, w573) -> (resulting string=w579:string)  [unwired: 2 in, 1 out]
            n307 = One Button Dialog(message=w579) -> ()  [unwired: 1 in, 1 out]
          }
          frame True {
            n308 = call "NextState.vi"("Data"="Waypoint upload verified." ("State"), "State"="Status", "Queue In"=w582) -> ()  [unwired: 7 in, 2 out]
            n309 = One Button Dialog(message="Waypoint upload successful!") -> ()  [unwired: 1 in, 1 out]
          }
        }
      }
      frame "--- File Storage ---" {
      }
      frame "Save Waypoints To File" {
        w586 = T5 0 items=["User Home"=0, "User Desktop"=1, "User Documents"=2, "User Application Data"=3, "User Preferences"=4, "User Temporary"=5, "Public Documents"=6, "Public Application Data"=7, "Public Preferences"=8, "Public Cache"=13, "System Core Libraries"=9, "System Installed Libraries"=10, "Application Files"=11, "Boot Volume Root"=12] ("system directory type")
        n310 = Unbundle By Name(w588) -> ("Waypoints"=w595:T1[])
        n311 = call <vilib>:"Get System Directory.vi"("system directory type"=w586) -> ("system directory"=w594:path)  [unwired: 10 in]
        n312 = call "File Dialog"("start path"=w594, "prompt"="Select location to store waypoint file:", "default name"="Waypoints", "pattern (all files)"="*.ini") -> ("selected path"=w591:path, "cancelled"=w592:bool)  [unwired: 8 in, 2 out]
        n313 = case shown="False" w592 {
          tunnel: w595 -> [w607 _]
          tunnel: w591 -> [w606 _]
          tunnel: w588 -> [w601 w635]
          tunnel: [w600 w635] -> w587
          frame False {
            n314 = call <vilib>:"Open Config Data.vi"("configuration file path"=w606) -> ("error out"=w604:errorcluster, "refnum"=w605:T6)  [unwired: 8 in, 1 out]
            n315 = for {
              tunnel: w607 -> [w620] mode=indexing
              tunnel: w605 -> [w615]
              shift-right: [w610] -> w603
              shift-left: w604 -> [w614]
              tunnel: [w609] -> w602
              i -> [w612]
              n316 = Unbundle By Name(w620) -> ("NS"=w634:u16, "LatD"=w632:dbl, "LatM"=w629:dbl, "LatS"=w628:dbl, "EW"=w625:u16, "LonD"=w623:dbl, "LonM"=w622:dbl, "LonS"=w621:dbl, "Alt"=w616:dbl)
              n317 = Greater Than 0?(x=w625) -> (x > 0?=w627:bool)
              n318 = Greater Than 0?(x=w634) -> (x > 0?=w633:bool)
              n319 = Negate(x=w632) -> (-x=w631:dbl)
              n320 = Negate(x=w623) -> (-x=w624:dbl)
              n321 = Select(t=w631, s=w633, f=w632) -> (s? t:f=w630:dbl)
              n322 = Select(t=w624, s=w627, f=w623) -> (s? t:f=w626:dbl)
              n323 = call "ConvertDMS2DD.vi"("Seconds"=w628, "Minutes"=w629, "Degrees"=w630) -> ("Degree Decimal"=w618:dbl)  [unwired: 7 in, 1 out]
              n324 = call "ConvertDMS2DD.vi"("Seconds"=w621, "Minutes"=w622, "Degrees"=w626) -> ("Degree Decimal"=w617:dbl)  [unwired: 7 in, 1 out]
              n325 = Format Into String(format string="%f,%f,%f", w618, w617, w616) -> (resulting string=w613:string)  [unwired: 2 in, 1 out]
              n326 = Number To Decimal String(number=w612) -> (decimal integer string=w611:string)  [unwired: 1 in]
              n327 = call-poly <vilib>:"Write Key.vi"("section"="Waypoints", "error in (no error)"=w614, "value"=w613, "key"=w611, "refnum"=w615) -> ("error out"=w610:errorcluster, "refnum out"=w609:T6)  [unwired: 4 in, 1 out]
            }
            n328 = call <vilib>:"Close Config Data.vi"("error in (no error)"=w603, "refnum"=w602) -> ("error out"=w599:errorcluster)  [unwired: 8 in, 1 out]
            n329 = Bundle By Name(cluster=w601, "Error"=w599) -> (w600:T2)
            n330 = Select(t="Error storing waypoints!", s=w599, f="Waypoints stored successfully.") -> (s? t:f=w596:string)
            n331 = One Button Dialog(message=w596) -> ()  [unwired: 1 in, 1 out]
          }
          frame True {
          }
        }
      }
      frame "Load Waypoints From File" {
        w637 = T5 0 items=["User Home"=0, "User Desktop"=1, "User Documents"=2, "User Application Data"=3, "User Preferences"=4, "User Temporary"=5, "Public Documents"=6, "Public Application Data"=7, "Public Preferences"=8, "Public Cache"=13, "System Core Libraries"=9, "System Installed Libraries"=10, "Application Files"=11, "Boot Volume Root"=12] ("system directory type")
        n332 = call <vilib>:"Get System Directory.vi"("system directory type"=w637) -> ("system directory"=w645:path)  [unwired: 10 in]
        n333 = call "File Dialog2"("start path"=w645, "prompt"="Select waypoint file:", "default name"="Waypoints", "pattern (all files)"="*.ini") -> ("selected path"=w642:path, "cancelled"=w643:bool)  [unwired: 8 in, 2 out]
        n334 = case shown="False" w643 {
          tunnel: w642 -> [w671 _]
          tunnel: w638 -> [w670 w720]
          tunnel: [w669 w720] -> w639
          tunnel: w636 -> [w657 _]
          frame False {
            w663 = "Waypoints" ("section")
            n335 = call <vilib>:"Open Config Data.vi"("configuration file path"=w671) -> ("error out"=w668:errorcluster, "refnum"=w667:T6)  [unwired: 8 in, 1 out]
            n336 = call <vilib>:"Get Key Names.vi"("section"=w663, "error in (no error)"=w668, "refnum"=w667) -> ("error out"=w666:errorcluster, "key names"=w664:string[], "refnum out"=w665:T6)  [unwired: 5 in, 1 out]
            n337 = for {
              tunnel: w664 -> [w716] mode=indexing
              tunnel: w665 -> [w718]
              shift-right: [w710] -> w661
              shift-left: w666 -> [w719]
              tunnel: w663 -> [w717]
              tunnel: [w715] -> w659 mode=indexing
              tunnel: [w709] -> w662
              tunnel: [w708] -> w658 mode=indexing
              n338 = call-poly <vilib>:"Read Key.vi"("section"=w717, "error in (no error)"=w719, "key"=w716, "refnum"=w718) -> ("error out"=w710:errorcluster, "value"=w713:string, "refnum out"=w709:T6)  [unwired: 4 in, 1 out]
              n339 = Decimal String To Number(string=w716) -> (number=w715:i32)  [unwired: 2 in, 1 out]
              n340 = Spreadsheet String To Array(delimiter (Tab)=",", format string="%f", spreadsheet string=w713) -> (array=w711:dbl[][])  [unwired: 1 in]
              n341 = Index Array(array=w711) -> (element=w708:dbl[])  [unwired: 2 in]
            }
            n342 = call "NextState.vi"("State"="Overall Waypoint Update", "Queue In"=w657) -> ("Queue Out"=w654:refnum<queue>)  [unwired: 8 in, 1 out]
            n343 = call "NextState.vi"("Data"=1000, "State"="Delay", "Queue In"=w654) -> ("Queue Out"=w653:refnum<queue>)  [unwired: 7 in, 1 out]
            n344 = call <vilib>:"Close Config Data.vi"("error in (no error)"=w661, "refnum"=w662) -> ("error out"=w655:errorcluster)  [unwired: 8 in, 1 out]
            n345 = Array Size(array=w659) -> (size(s)=w660:i32)
            n346 = for {
              N: w660 -> [_]
              tunnel: w659 -> [w707]
              tunnel: w658 -> [w706]
              tunnel: [w684] -> w646 mode=indexing
              i -> [w683]
              w703 = FALSE ("Type")
              w702 = u16 1 items=["E", "W"] ("EW")
              w701 = u16 0 items=["E", "W"] ("EW")
              w696 = u16 1 items=["N", "S"] ("NS")
              w695 = u16 0 items=["N", "S"] ("NS")
              n347 = Search 1D Array(1D array=w707, element=w683) -> (index of element=w705:i32)  [unwired: 1 in]
              n348 = Index Array(array=w706, index (row)=w705) -> (element=w704:dbl[])  [unwired: 1 in]
              n349 = Index Array(array=w704) -> (element #1=w686:dbl, element #2=w687:dbl, element #3=w688:dbl)  [unwired: 3 in]
              n350 = call "ConvertDD2DMS.vi"("Type"=w703, "Degree Decimal"=w686) -> ("Seconds"=w691:dbl, "Minutes"=w690:dbl, "Degrees"=w689:dbl, "NE?"=w694:bool)  [unwired: 5 in, 1 out]
              n351 = call "ConvertDD2DMS.vi"("Type"=w703, "Degree Decimal"=w687) -> ("Seconds"=w693:dbl, "Minutes"=w692:dbl, "Degrees"=w698:dbl, "NE?"=w699:bool)  [unwired: 5 in, 1 out]
              n352 = Select(t=w695, s=w694, f=w696) -> (s? t:f=w697:u16)
              n353 = Select(t=w701, s=w699, f=w702) -> (s? t:f=w700:u16)
              n354 = Bundle By Name(cluster=T1 {"LatD"=0.0, "LatM"=0.0, "LatS"=0.0, "LonD"=0.0, "LonM"=0.0, "LonS"=0.0, "Alt"=0.0, "NS"=0, "EW"=0} ("Waypoint"), "LatD"=w689, "LatM"=w690, "LatS"=w691, "NS"=w697, "LonD"=w698, "LonM"=w692, "LonS"=w693, "EW"=w700, "Alt"=w688) -> (w684:T1)
            }
            n355 = case shown="No Error" w655 {
              tunnel: w653 -> [w675 _]
              frame No Error {
                n356 = Two Button Dialog(message="Would you also like to upload these waypoints to the AeroQuad?", 1:"Later" ("F button name (\"Cancel\")")) -> (T button?=w674:bool)  [unwired: 1 in]
                n357 = case shown="True" w674 {
                  tunnel: w675 -> [w678 w681]
                  tunnel: [w678 w679] -> w672
                  frame False {
                  }
                  frame True {
                    n358 = call "NextState.vi"("State"="Upload Waypoints", "Queue In"=w681) -> ("Queue Out"=w679:refnum<queue>)  [unwired: 8 in, 1 out]
                  }
                }
                n359 = call "NextState.vi"("State"="Center Map", "Queue In"=w672) -> ()  [unwired: 8 in, 2 out]
              }
              frame Error {
                n360 = One Button Dialog(message="Error loading waypoints!") -> ()  [unwired: 1 in, 1 out]
              }
            }
            n361 = local write "Waypoint List"(w646) -> ()
            n362 = Array Size(array=w646) -> (size(s)=w647:i32)
            n363 = Bundle By Name(cluster=w670, "Error"=w655, "Waypoints"=w646) -> (w669:T2)
            n364 = Subtract(x=w647, y=3) -> (x-y=w649:i32)
            n365 = Build Array(w649) -> (w650:i32[])
            n366 = property on="Waypoint List" class="Arr (strict)"("Index Values"=w650) -> ()  [unwired: 2 in, 2 out]
          }
          frame True {
          }
        }
      }
      frame "--- Vehicle Position ---" {
      }
      frame "Vehicle Telemetry" {
        n367 = Variant To Data(Variant=w724, type=FALSE) -> (data=w722:bool)  [unwired: 1 in, 1 out]
        n368 = Unbundle By Name(w727) -> ("GUIQueue"=w725:refnum<queue>)  [unwired: 1 out]
        n369 = case shown="False" w722 {
          tunnel: w727 -> [w737 w749]
          tunnel: [w735 w748] -> w726
          tunnel: w725 -> [w733 w741]
          frame True {
            n370 = call "LookupCommands.vi"("CommandName"="Telemetry") -> ("CommandValue"=w729:string)  [unwired: 10 in]
            n371 = call "NextState.vi"("Data"=w729, "State"="Request Telemetry", "Queue In"=w733) -> ("Error Out"=w731:errorcluster, "Queue Out"=w732:refnum<queue>)  [unwired: 7 in]
            n372 = call "NextState.vi"("Error In"=w731, "State"="Read Integers Continuous", "Queue In"=w732) -> ("Error Out"=w736:errorcluster)  [unwired: 7 in, 1 out]
            n373 = Bundle By Name(cluster=w737, "TlmType"="Update Vehicle Telemetry", "Error"=w736) -> (w735:T2)
          }
          frame False {
            n374 = call "NextState.vi"("State"="Clear Queue", "Queue In"=w741) -> ("Queue Out"=w740:refnum<queue>)  [unwired: 8 in, 1 out]
            n375 = call "NextState.vi"("State"="Clear Serial Comm", "Queue In"=w740) -> ("Queue Out"=w739:refnum<queue>)  [unwired: 8 in, 1 out]
            n376 = call "LookupCommands.vi"("CommandName"="StopTelem") -> ("CommandValue"=w745:string)  [unwired: 10 in]
            n377 = call "NextState.vi"("Data"=w745, "State"="Request Telemetry", "Queue In"=w739) -> ("Error Out"=w744:errorcluster)  [unwired: 7 in, 1 out]
            n378 = Bundle By Name(cluster=w749, "Error"=w744) -> (w748:T2)
          }
        }
      }
      frame "Update Vehicle Telemetry" {
        w750 = FALSE
        # "0 State\n1 Lat\n2 Lon\n3 Height\n4 Course\n5 Speed\n6 Accuracy\n7 Sats"
        n379 = Unbundle By Name(w756) -> ("Data"=w755:i32[][])
        n380 = Index Array(array=w755) -> (element=w754:i32[])  [unwired: 2 in]
        n381 = for {
          tunnel: w754 -> [w763] mode=indexing
          i -> [w764]
          n382 = case shown="4" w764 {
            tunnel: w763 -> [_ _ w766 w769 w772 w776 w778 w780 w782]
            frame Default {
            }
            frame 0 {
            }
            frame 1 {
              n383 = Divide(x=w766, y=10000000.0) -> (x/y=w765:dbl)
              n384 = local write "Latitude"(w765) -> ()
            }
            frame 2 {
              n385 = Divide(x=w769, y=10000000.0) -> (x/y=w768:dbl)
              n386 = local write "Longitude"(w768) -> ()
            }
            frame 3 {
              n387 = Divide(x=w772, y=10.0) -> (x/y=w771:dbl)
              n388 = local write "Altitude"(w771) -> ()
            }
            frame 4 {
              n389 = To Word Integer(number=w776) -> (16bit integer=w775:i16)
              n390 = local write "Course"(w775) -> ()
              n391 = local write "Heading"(w775) -> ()
              n392 = Bundle(w775, w775) -> (w774:cluster{i16, i16})  [unwired: 1 in]
              n393 = local write "Compass"(w774) -> ()
            }
            frame 5 {
              n394 = To Unsigned Byte Integer(number=w778) -> (unsigned 8bit integer=w777:u8)
              n395 = local write "Speed"(w777) -> ()
            }
            frame 6 {
              n396 = To Unsigned Word Integer(number=w780) -> (unsigned 16bit integer=w779:u16)
              n397 = local write "HDOP"(w779) -> ()
            }
            frame 7 {
              n398 = To Unsigned Word Integer(number=w782) -> (unsigned 16bit integer=w781:u16)
              n399 = local write "Sat Count"(w781) -> ()
            }
          }
        }
        n400 = local read "Update Rate"() -> (w752:dbl)
        n401 = call "Elapsed Time2"("Time Target (s)"=w752) -> ("Time has Elapsed"=w751:bool)  [unwired: 11 in, 7 out]
        n402 = case shown="True" w751 {
          tunnel: w753 -> [_ w762]
          frame False {
          }
          frame True {
            # "Update map every second."
            n403 = local read "Longitude"() -> (w758:dbl)
            n404 = local read "Latitude"() -> (w757:dbl)
            n405 = Format Into String(format string="%.7f,%7f", w757, w758) -> (resulting string=w759:string)  [unwired: 2 in, 1 out]
            n406 = call "NextState.vi"("Data"=w759, "State"="Set Vehicle Position", "Queue In"=w762) -> ()  [unwired: 7 in, 2 out]
          }
        }
        n407 = property on="Current" class="DigNum (strict)"("Visible"=w750) -> ()  [unwired: 2 in, 2 out]
        n408 = property on="Capacity" class="DigNum (strict)"("Visible"=w750) -> ()  [unwired: 2 in, 2 out]
        n409 = property on="Voltage" class="DigNum (strict)"("Visible"=w750) -> ()  [unwired: 2 in, 2 out]
        n410 = property on="RSSI" class="Slide (strict)"("Visible"=w750) -> ()  [unwired: 2 in, 2 out]
        n411 = property on="Battery" class="Slide (strict)"("Visible"=w750) -> ()  [unwired: 2 in, 2 out]
      }
      frame "Set Vehicle Position" {
        n412 = Unbundle By Name(w790) -> ("Map"=w789:refnum<k7>, "Internet"=w783:bool)
        n413 = Variant To Data(Variant=w785, type=w786) -> (data=w784:string)  [unwired: 1 in, 1 out]
        n414 = Format Into String(format string="javascript:updateVehiclePosition(%s,1);" ("URL"), w784) -> (resulting string=w787:string)  [unwired: 2 in, 1 out]
        n415 = call "WaitForBrowser.vi"("Connection"=w783, "BrowserCommand"=w787, "BrowserRef"=w789) -> ()  [unwired: 7 in, 2 out]
      }
    }
  }
  n416 = while {
    tunnel: w8 -> [w798]
    tunnel: w2 -> [w797]
    tunnel: w1 -> [w796]
    stop <- w792 stop-if-true
    n417 = Dequeue Element(queue=w797, timeout in ms (-1)=1000, error in (no error)=w796) -> (queue out=w791:refnum<queue>, element=w794:string, error out=w795:errorcluster)  [unwired: 1 out]
    n418 = case shown="Default" w794 {
      selector: w794 -> [w814 _ w867]
      tunnel: w798 -> [w810 _ _]
      tunnel: w795 -> [_ w861 _]
      tunnel: [FALSE _ _] -> w792
      tunnel: w791 -> [_ w860 _]
      frame Default {
        w816 = 32  # Frame Size
        n419 = call "ModemTelemetryParser.vi"("Frame Size"=w816, "Serial Data In"=w814) -> ("Valid"=w799:bool, "Detected Frames"=w815:u8[][])  [unwired: 7 in, 1 out]
        n420 = for {
          tunnel: w815 -> [w859] mode=indexing
          tunnel: [w854] -> w811
          tunnel: [w853] -> w812
          w856 = 10000000.0
          n421 = call "ModemTelemetryDecode.vi"("Encoded Data"=w859) -> ("TelemetryPacket"=w858:T8)  [unwired: 9 in, 1 out]
          n422 = Unbundle By Name(w858) -> ("latitude"=w857:i32, "longitude"=w855:i32, "altitude"=w847:i16, "course"=w838:i16, "heading"=w845:i16, "speed"=→"Speed":u8, "voltage"=w851:u8, "current"=→"Current":u8, "capacity"=→"Capacity":u16, "RSSI"=→"RSSI":u8, "reserved"=w833:u16)  [unwired: 1 out]
          "Course" <- w838
          n423 = Compound Arithmetic op=ADD(i16 360 ("value"), w845) -> (w844:i16)
          n424 = Logical Shift(y=i8 -12, x=w833) -> (x << y=→"Sat Count":u16)
          n425 = Compound Arithmetic op=AND(w833, u16 4095 ("value")) -> (→"HDOP":u16)
          n426 = Less Than 0?(x=w845) -> (x < 0?=w846:bool)
          n427 = Select(t=w844, s=w846, f=w845) -> (s? t:f=w839:i16)
          "Heading" <- w839
          n428 = Bundle("heading"=w839, "course"=w838) -> (→"Compass":cluster{"heading":i16, "course":i16})  [unwired: 1 in]
          n429 = Divide(x=w847, y=10.0) -> (x/y=→"Altitude":dbl)
          n430 = Divide(x=w851, y=10.0 ("x/y")) -> (x/y=→"Voltage" →"Battery":dbl)
          n431 = Divide(x=w857, y=w856) -> (x/y=w854:dbl)
          "Latitude" <- w854
          n432 = Divide(x=w855, y=w856) -> (x/y=w853:dbl)
          "Longitude" <- w853
        }
        n433 = case shown="True" w799 {
          frame False {
          }
          frame True {
            w817 = TRUE
            n434 = property on="Voltage" class="DigNum (strict)"("Visible"=w817) -> ()  [unwired: 2 in, 2 out]
            n435 = property on="Current" class="DigNum (strict)"("Visible"=w817) -> ()  [unwired: 2 in, 2 out]
            n436 = property on="Battery" class="Slide (strict)"("Visible"=w817) -> ()  [unwired: 2 in, 2 out]
            n437 = property on="RSSI" class="Slide (strict)"("Visible"=w817) -> ()  [unwired: 2 in, 2 out]
            n438 = property on="Capacity" class="DigNum (strict)"("Visible"=w817) -> ()  [unwired: 2 in, 2 out]
          }
        }
        n439 = call "Elapsed Time"("Time Target (s)"="Update Rate") -> ("Time has Elapsed"=w805:bool)  [unwired: 11 in, 7 out]
        n440 = property on="Battery" class="Slide (strict)"() -> ("Value"=w809:dbl)  [unwired: 2 in, 2 out]
        n441 = property on="RSSI" class="Slide (strict)"() -> ("Value"=w801:u8)  [unwired: 2 in, 2 out]
        n442 = Compound Arithmetic op=AND(w805, w799) -> (w804:bool)
        n443 = Multiply(x=w809, y=100.0) -> (x*y=w807:dbl)
        n444 = case shown="True" w804 {
          tunnel: w812 -> [_ w828]
          tunnel: w811 -> [_ w829]
          tunnel: w810 -> [_ w827]
          frame False {
          }
          frame True {
            # "Update map every second."
            n445 = Format Into String(format string="%.7f,%7f", w829, w828) -> (resulting string=w825:string)  [unwired: 2 in, 1 out]
            n446 = call "NextState.vi"("Data"=w825, "State"="Set Vehicle Position", "Queue In"=w827) -> ()  [unwired: 7 in, 2 out]
          }
        }
        n447 = case shown="951..1000" w807 {
          tunnel: [u32 16768256 u32 6618880 u32 16711680] -> w806
          frame 951..1000 {
          }
          frame Default {
          }
          frame ..950 {
          }
        }
        n448 = case shown="0..25" w801 {
          tunnel: [u32 16768256 u32 6618880 u32 16711680] -> w802
          tunnel: [_ _ TRUE] -> w800
          frame 26..50 {
          }
          frame Default {
          }
          frame 0..25 {
          }
        }
        n449 = property on="Battery" class="Slide (strict)"("Fill Color"=w806) -> ()  [unwired: 2 in, 2 out]
        n450 = property on="RSSI" class="Slide (strict)"("Fill Color"=w802, "Blinking"=w800) -> ()  [unwired: 2 in, 2 out]
      }
      frame "***Disconnect***" {
        (unwired) T8 {"id"=0, "latitude"=0, "longitude"=0, "altitude"=0, "course"=0, "heading"=0, "speed"=0, "voltage"=0, "current"=0, "capacity"=0, "reserved"=0, "ecc"=[], "RSSI"=0}  # TelemetryPacket
        n451 = Flush Queue(queue=w860, error in (no error)=w861) -> ()  [unwired: 3 out]
      }
      frame "Fresh Data", "Stale Data" {
        n452 = Equal?(x=w867, y="Fresh Data") -> (x = y?=w864:bool)
        n453 = Select(t=T7."Enabled" ("Disabled"), s=w864, f=T7."Disabled and Grayed Out" ("Disabled")) -> (s? t:f=w862:T7)
        n454 = property on="Latitude" class="DigNum (strict)"("DisabledEnum"=w862) -> ()  [unwired: 2 in, 2 out]
        n455 = property on="Longitude" class="DigNum (strict)"("DisabledEnum"=w862) -> ()  [unwired: 2 in, 2 out]
        n456 = property on="Altitude" class="DigNum (strict)"("DisabledEnum"=w862) -> ()  [unwired: 2 in, 2 out]
        n457 = property on="Compass" class="Knob (strict)"("DisabledEnum"=w862) -> ()  [unwired: 2 in, 2 out]
        n458 = property on="Capacity" class="DigNum (strict)"("DisabledEnum"=w862) -> ()  [unwired: 2 in, 2 out]
        n459 = property on="RSSI" class="Slide (strict)"("DisabledEnum"=w862) -> ()  [unwired: 2 in, 2 out]
        n460 = property on="Heading" class="DigNum (strict)"("DisabledEnum"=w862) -> ()  [unwired: 2 in, 2 out]
        n461 = property on="Course" class="DigNum (strict)"("DisabledEnum"=w862) -> ()  [unwired: 2 in, 2 out]
        n462 = property on="Battery" class="Slide (strict)"("DisabledEnum"=w862) -> ()  [unwired: 2 in, 2 out]
        n463 = property on="Speed" class="DigNum (strict)"("DisabledEnum"=w862) -> ()  [unwired: 2 in, 2 out]
        n464 = property on="Current" class="DigNum (strict)"("DisabledEnum"=w862) -> ()  [unwired: 2 in, 2 out]
        n465 = property on="Voltage" class="DigNum (strict)"("DisabledEnum"=w862) -> ()  [unwired: 2 in, 2 out]
        n466 = property on="Course" class="ColBox"("DisabledEnum"=w862) -> ()  [unwired: 2 in, 2 out]
        n467 = property on="Heading" class="ColBox"("DisabledEnum"=w862) -> ()  [unwired: 2 in, 2 out]
      }
    }
  }
  n468 = while {
    tunnel: w8 -> [w868]
    stop <- w869 stop-if-true
    n469 = event shown="[18] \"VehicleUpdate\": Value Change" {
      selector: _ -> [_ _ _ _ _ _ _ _ _ _ _ _ _ _ _ _ _ _ _ _]
      dyn-events: _ -> [_ _ _ _ _ _ _ _ _ _ _ _ _ _ _ _ _ _ _ _]
      timeout: _ -> [_ _ _ _ _ _ _ _ _ _ _ _ _ _ _ _ _ _ _ _]
      tunnel: [FALSE _ _ _ _ _ _ _ _ _ _ _ _ _ _ _ _ _ _ TRUE] -> w869
      tunnel: w868 -> [w871 w875 w879 w881 w882 w884 _ _ w888 w891 _ w893 w897 w899 w901 w903 w904 _ w918 w920]
      event "Map": Mouse Down {
        # "Map->Mouse Down"
        n470 = event-data() -> ()  [unwired: 1 in, 1 out]
        n471 = call "NextState.vi"("State"="Process Waypoint List", "Queue In"=w871) -> ("Queue Out"=w870:refnum<queue>)  [unwired: 8 in, 1 out]
        n472 = call "NextState.vi"("State"="Request Waypoint Update", "Queue In"=w870) -> ()  [unwired: 8 in, 2 out]
      }
      event "Map": Mouse Enter {
        # "Map -> Mouse Enter"
        n473 = event-data() -> ()  [unwired: 1 in, 1 out]
        n474 = call "PriorityState.vi"("Data"="Click on map to select waypoints." ("State"), "State"="Send Status Message", "Queue In"=w875) -> ()  [unwired: 7 in, 2 out]
      }
      event "Recall": Value Change {
        n475 = event-data() -> ()  [unwired: 1 in, 1 out]
        n476 = call "PriorityState.vi"("State"="Recall Waypoints", "Queue In"=w879) -> ()  [unwired: 8 in, 2 out]
      }
      event "Delete": Value Change {
        n477 = event-data() -> ()  [unwired: 1 in, 1 out]
        n478 = call "NextState.vi"("State"="Clear Last Waypoint", "Queue In"=w881) -> ()  [unwired: 8 in, 2 out]
      }
      event "Upload": Value Change {
        n479 = event-data() -> ()  [unwired: 1 in, 1 out]
        n480 = call "NextState.vi"("State"="Upload Waypoints", "Queue In"=w882) -> ()  [unwired: 8 in, 2 out]
      }
      event "Clear": Value Change {
        n481 = event-data() -> ()  [unwired: 1 in, 1 out]
        n482 = call "NextState.vi"("State"="Clear Waypoint List", "Queue In"=w884) -> ()  [unwired: 8 in, 2 out]
      }
      event "Up": Value Change {
        n483 = event-data() -> ()  [unwired: 1 in, 1 out]
      }
      event "Down": Value Change {
        n484 = event-data() -> ()  [unwired: 1 in, 1 out]
      }
      event "ManualAdd": Value Change {
        n485 = event-data() -> ()  [unwired: 1 in, 1 out]
        n486 = call "NextState.vi"("State"="Process Waypoint List", "Queue In"=w888) -> ("Queue Out"=w887:refnum<queue>)  [unwired: 8 in, 1 out]
        n487 = call "NextState.vi"("State"="Overall Waypoint Update", "Queue In"=w887) -> ()  [unwired: 8 in, 2 out]
      }
      event "Home": Value Change {
        n488 = event-data() -> ()  [unwired: 1 in, 1 out]
        n489 = call "PriorityState.vi"("State"="Set Home Position", "Queue In"=w891) -> ()  [unwired: 8 in, 2 out]
      }
      event "NoFly": Value Change {
        n490 = event-data() -> ()  [unwired: 1 in, 1 out]
        n491 = One Button Dialog(message="This will be implemented in the next version.") -> ()  [unwired: 1 in, 1 out]
      }
      event "Waypoint List": Mouse Enter {
        n492 = event-data() -> ()  [unwired: 1 in, 1 out]
        n493 = call "PriorityState.vi"("Data"="Select \"Manual Update\" to update map with new waypoint info." ("State"), "State"="Send Status Message", "Queue In"=w893) -> ()  [unwired: 7 in, 2 out]
      }
      event "Waypoint List": Value Change {
        n494 = event-data() -> ()  [unwired: 1 in, 1 out]
        n495 = call "NextState.vi"("State"="Process Waypoint List", "Queue In"=w897) -> ()  [unwired: 8 in, 2 out]
      }
      event "Load": Value Change {
        n496 = event-data() -> ()  [unwired: 1 in, 1 out]
        n497 = call "NextState.vi"("State"="Load Waypoints From File", "Queue In"=w899) -> ()  [unwired: 8 in, 2 out]
      }
      event "Save": Value Change {
        n498 = event-data() -> ()  [unwired: 1 in, 1 out]
        n499 = call "NextState.vi"("State"="Save Waypoints To File", "Queue In"=w901) -> ()  [unwired: 8 in, 2 out]
      }
      event "Center": Value Change {
        n500 = event-data() -> ()  [unwired: 1 in, 1 out]
        n501 = call "NextState.vi"("State"="Center Map", "Queue In"=w903) -> ()  [unwired: 8 in, 2 out]
      }
      event "Slider": Value Change {
        n502 = event-data() -> ()  [unwired: 1 in, 1 out]
        n503 = call "NextState.vi"("State"="Move Slider", "Queue In"=w904) -> ()  [unwired: 8 in, 2 out]
      }
      event Mouse Move {
        n504 = event-data() -> ("SplitterRef"=w911:refnum<vi>)  [unwired: 1 in, 1 out]
        n505 = property on="Slider" class="Bool"() -> ("Width"=w909:u32)  [unwired: 2 in, 2 out]
        n506 = Increment(x=w909) -> (x+1=w906:u32)
        n507 = property class="Splitter"(reference=w911) -> (reference out=w908:refnum<vi>, "Position"=w910:i32)  [unwired: 1 in, 1 out]
        n508 = Less?(x=w910, y=w906) -> (x < y?=w907:bool)
        n509 = case shown="True" w907 {
          tunnel: w908 -> [_ w913]
          tunnel: w906 -> [_ w912]
          frame False {
          }
          frame True {
            n510 = property class="Splitter"(reference=w913, "Position"=w912) -> ()  [unwired: 1 in, 2 out]
          }
        }
      }
      event "VehicleUpdate": Value Change {
        n511 = event-data() -> ()  [unwired: 1 in, 1 out]
        n512 = feedback #1(FALSE) -> (w915:bool)
        n513 = Not(x=w915) -> (.not. x?=w914:bool)
        "VehiclePositionState" <- w914
        n514 = feedback-in #1(w914) -> ()
        n515 = call "NextState.vi"("Data"=w914, "State"="Vehicle Telemetry", "Queue In"=w918) -> ()  [unwired: 7 in, 2 out]
      }
      event Panel Close? {
        n516 = event-data() -> ()  [unwired: 1 in, 1 out]
        n517 = call "NextState.vi"("State"="Shutdown", "Queue In"=w920) -> ()  [unwired: 8 in, 2 out]
        n518 = event-data("Discard?"=TRUE) -> ()  [unwired: 1 in, 1 out]
      }
    }
  }
